vi "test.vi"() -> ()   [LabVIEW 2017]
uses:
  Measurement Utility/API/TestStand API.lvlib
panel:
  out "error out 4":errorcluster
  out "error out 3":errorcluster
  out "error out 2":errorcluster
  out "error out":errorcluster
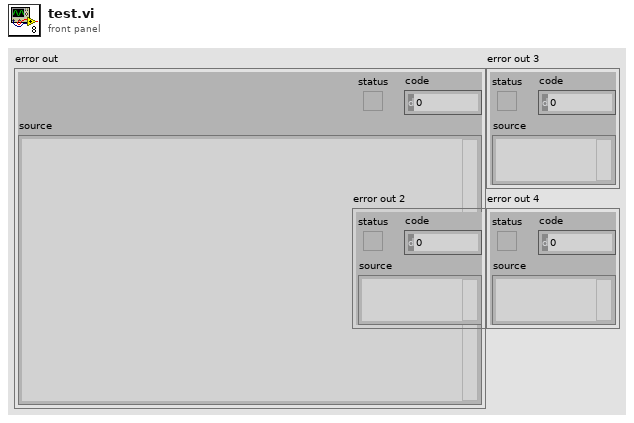
[diagram p1: front panel]
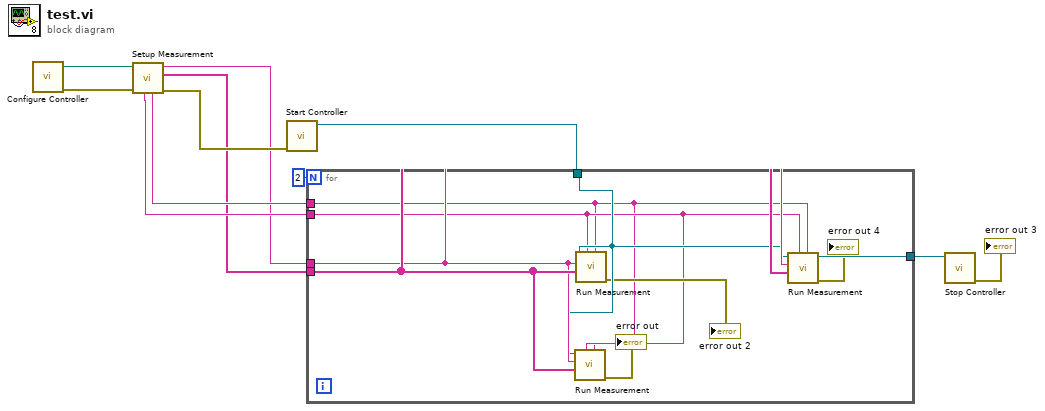
[diagram p0: block diagram]
diagram:
  n1 = call "Configure Controller.vi"() -> ("error IO"=w4:errorcluster, "Absolute Path"=w5:path)  [unwired: 10 in]
  n2 = call "Setup Measurement.vi"("error in (no error)"=w4, "Config File Path"=w5) -> ("error out"=w11:errorcluster, "Device Names"=w8:string[], "Measurement Name"=w2:string, "Array of Device Configuration"=w10:string, "Step Configuration"=w9:string)  [unwired: 4 in, 1 out]
  n3 = call "Start Controller.vi"("error in (no error)"=w11) -> ("Controller Queue"=w6:refnum<class "Message Enqueuer.lvclass">)  [unwired: 8 in, 2 out]
  n4 = for {
    N: 2 -> [_]
    tunnel: w10 -> [w12]
    tunnel: w9 -> [w13]
    tunnel: w2 -> [w18]
    tunnel: w8 -> [w19]
    tunnel: w6 -> [w17]
    tunnel: [w20] -> w7
    n5 = call "Run Measurement.vi"("Array of Device Configuration"=w12, "Step Configuration"=w13, "Device Names"=w19, "Measurement Name"=w18, "Self Enqueuer In"=w17) -> ("error out"=→"error out":errorcluster)  [unwired: 4 in, 2 out]
    n6 = call "Run Measurement.vi"("Array of Device Configuration"=w12, "Step Configuration"=w13, "Device Names"=w19, "Measurement Name"=w18, "Self Enqueuer In"=w17) -> ("error out"=→"error out 2":errorcluster)  [unwired: 4 in, 2 out]
    n7 = call "Run Measurement.vi"("Array of Device Configuration"=w12, "Step Configuration"=w13, "Device Names"=w19, "Measurement Name"=w18, "Self Enqueuer In"=w17) -> ("error out"=→"error out 4":errorcluster, "Self Enqueuer Out"=w20:refnum<class "Message Enqueuer.lvclass">)  [unwired: 4 in, 1 out]
  }
  n8 = call "Stop Controller.vi"("TestStand Controller Queue"=w7) -> ("error out"=→"error out 3":errorcluster)  [unwired: 10 in]
